vi "SourceMeterF.vi"() -> ()   [LabVIEW 2017]
uses:
  <vilib>/express/express signal manip/GetorSetDDTAttributes/Set DDT Attributes/Set DDT Properties.xnode
  <vilib>/express/express shared/transition.llb/Dynamic To Waveform Array.vi
  <vilib>/express/express signal manip/GetorSetDDTAttributes/Set DDT Attributes/SetT0.vi
  <vilib>/express/express shared/transition.llb/Waveform Array To Dynamic.vi
  <vilib>/express/express signal manip/GetorSetDDTAttributes/Set DDT Attributes/sub Set StartTimeStamp.vi
  <vilib>/express/express signal manip/GetorSetDDTAttributes/Set DDT Attributes/Set DDT Attributes.lvlib
panel:
  in  "?":bool
  in  "Registerkarte":T1(tab)
  in  "VISA resource name":refnum<visa-resource-name>
  in  "Script Name":string="myscript"
  in  "Save script (No)":bool
  in  "Load Options (Load)":enum16{"Load", "Load & Run"}(ring)
  in  "Filename":path caption="File name"
  in  "Save Data":bool
  in  "U / V":dbl=10.0
  in  "I /A":dbl=0.5
  in  "Q /C":dbl=1.0
  in  "Script":string
  out "Nr. of Measurments":i32
  out "Saving Data":bool
  out "C":dbl
  out "A":dbl
  out "V":dbl
  out "thresholdC":bool
  out "thresholdI":bool
  out "Graph":cluster{dbl, "Numerisch":dbl, "Numerisch 3":dbl}(graph)
  out "current/charge":cluster{dbl[], dbl[]}[](graph) caption="XY-Graph"
  out "Voltage":cluster{dbl[], dbl[]}(graph) caption="XY-Graph"
  out "error out 2":errorcluster
  out "current":dbl
  out "charge":dbl
  out "voltage":dbl
  out "delay1":u32
  out "delay loop2":dbl
  out "Elementanzahl in Queue":i32(slide) scale=0.0..10000.0
  # "Threshold"
  # "total time (ms)"
  # "Threshold"
  # "Threshold!"
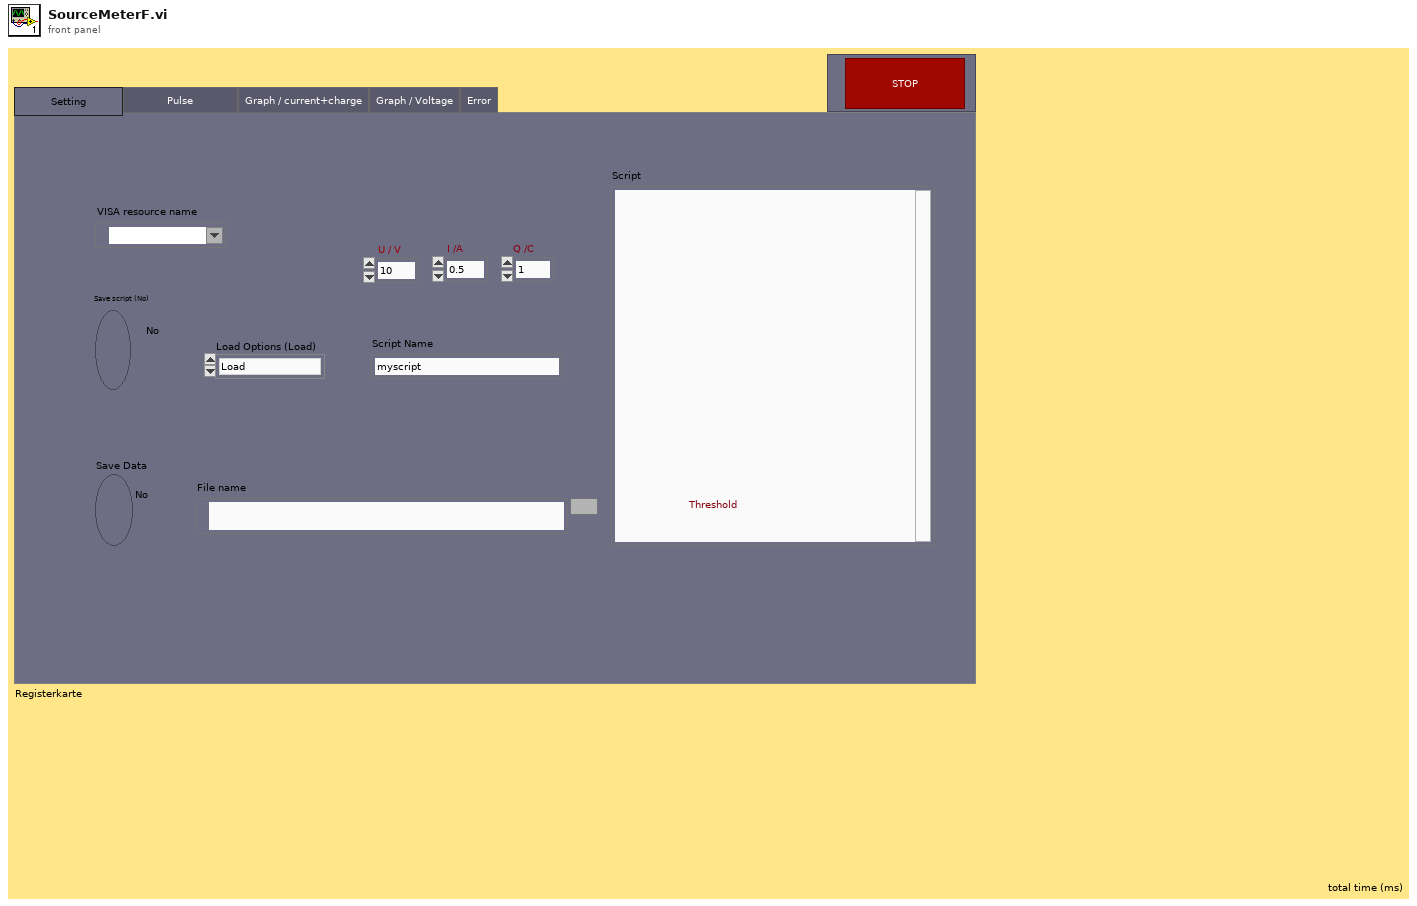
[diagram p1: front panel]
types:
  T1 = enum32{"Setting                    ", "Pulse                         ", "Graph / current+charge", "Graph / Voltage", "Error"}
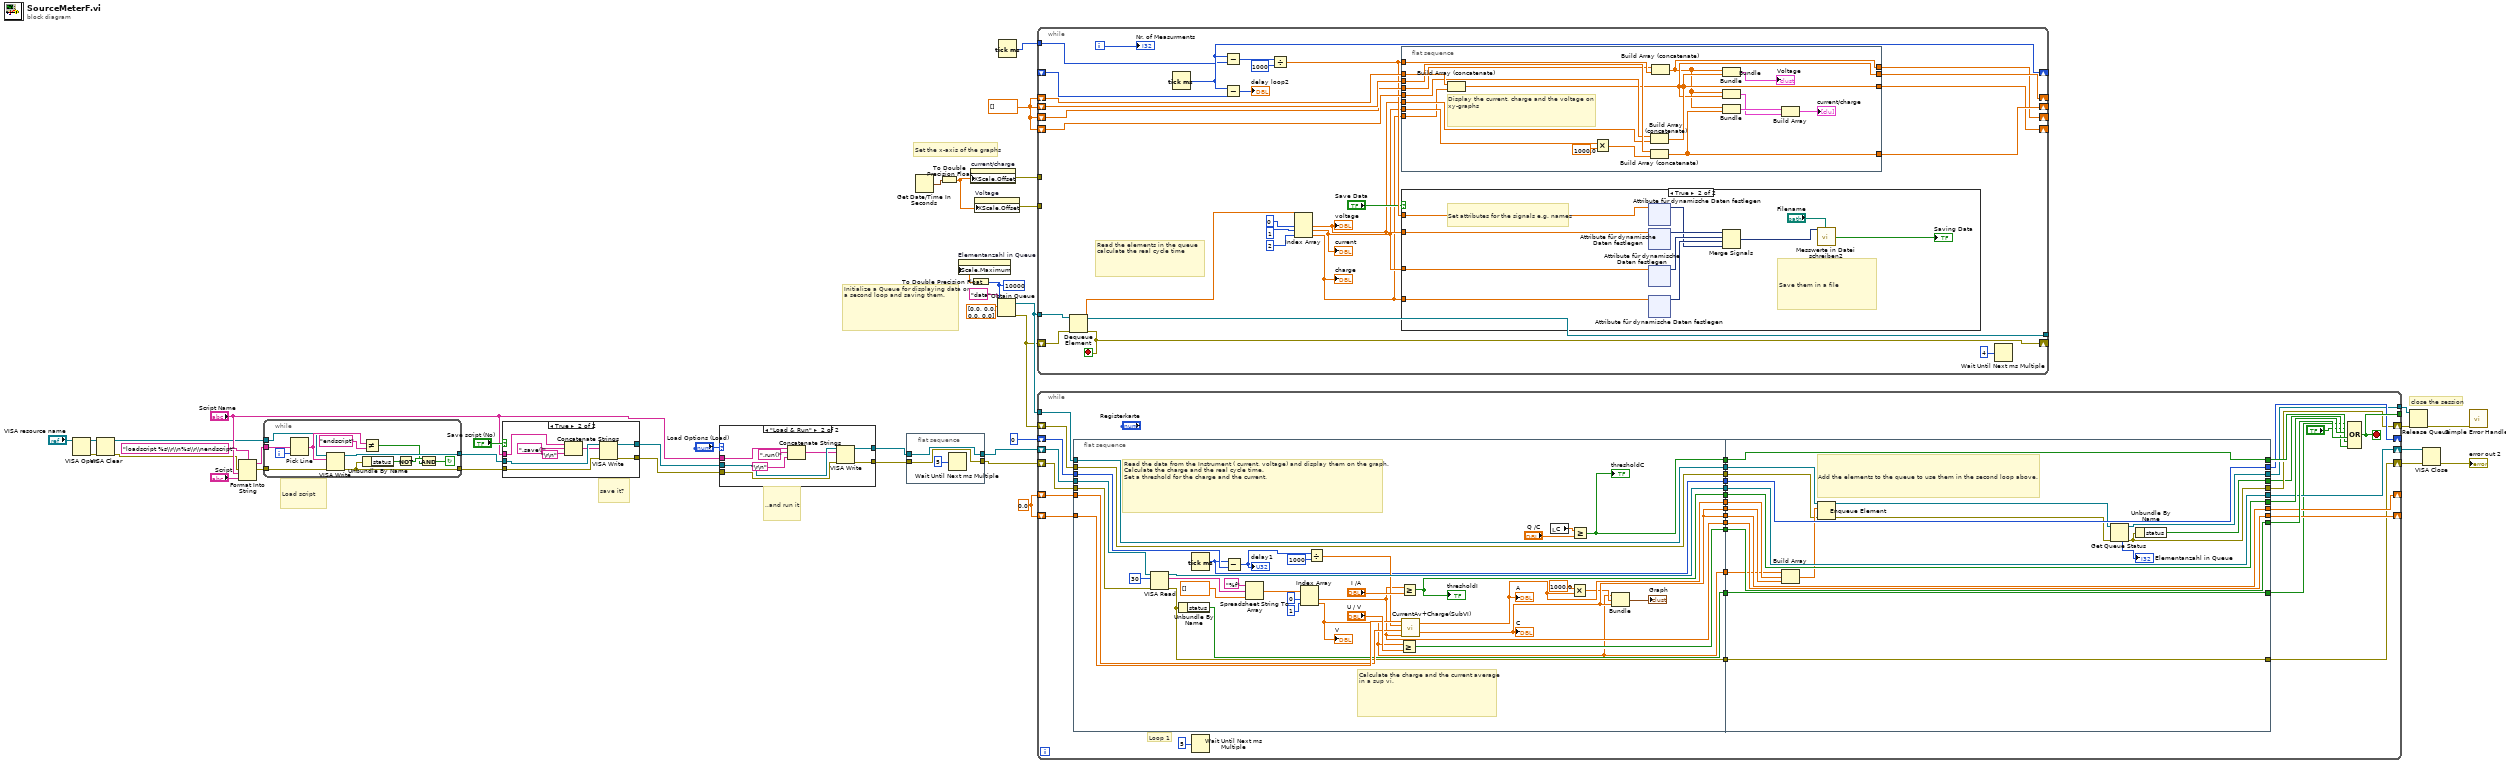
[diagram p0: block diagram]
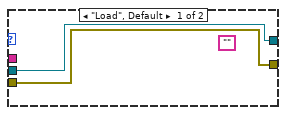
[diagram p2: hidden frame]
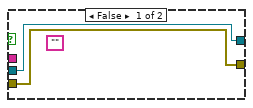
[diagram p3: hidden frame]
diagram:
  w23 = 10000 ("Maximale Queue-Größe (-1, unbegrenzt)")
  w24 = dbl[] []
  w33 = 0.0 ("Numerisch")
  # "close the session"
  # "Initialize a Queue for displaying data on a second loop and saving them."
  # "Set the x-axis of the graphs"
  # "..and run it"
  # "save it?"
  # "Load script"
  n1 = VISA Open(VISA resource name="VISA resource name") -> (VISA resource name=w20:refnum<visa-resource-name>, error out=w21:errorcluster)  [unwired: 4 in]
  n2 = VISA Clear(VISA resource name=w20, error in (no error)=w21) -> (VISA resource name out=w2:refnum<visa-resource-name>, error out=w3:errorcluster)
  n3 = Format Into String(format string="loadscript %s\\r\\n%s\\r\\nendscript", error in=w3, "Script Name", "Script") -> (resulting string=w6:string, error out=w15:errorcluster)  [unwired: 1 in]
  n4 = while {
    tunnel: w15 -> [w49]
    tunnel: [w46] -> w12
    tunnel: [w48] -> w11
    tunnel: w6 -> [w47]
    tunnel: w2 -> [w41]
    i -> [w51]
    stop <- w45 continue-if-true
    n5 = Pick Line(multi-line string=w47, line index=w51) -> (output string=w50:string)  [unwired: 1 in]
    n6 = VISA Write(VISA resource name=w41, write buffer=w50, error in (no error)=w49) -> (VISA resource name out=w48:refnum<visa-resource-name>, error out=w46:errorcluster)  [unwired: 1 out]
    n7 = Unbundle By Name(w46) -> ("status"=w44:bool)
    n8 = Not Equal?(x=w50, y="endscript") -> (x != y?=w42:bool)
    n9 = Not(x=w44) -> (.not. x?=w43:bool)
    n10 = And(x=w43, y=w42) -> (x .and. y?=w45:bool)
  }
  n11 = case shown="True" "Save script (No)" {
    tunnel: w12 -> [w53 w61]
    tunnel: w11 -> [w54 w62]
    tunnel: "Script Name" -> [_ w59]
    tunnel: [w54 w58] -> w9
    tunnel: [w53 w57] -> w8
    frame False {
      (unwired) ""
    }
    frame True {
      n12 = Concatenate Strings(w59, ".save()" ("string"), "\r\n") -> (w56:string)
      n13 = VISA Write(VISA resource name=w62, write buffer=w56, error in (no error)=w61) -> (VISA resource name out=w58:refnum<visa-resource-name>, error out=w57:errorcluster)  [unwired: 1 out]
    }
  }
  n14 = case shown="\"Load & Run\"" "Load Options (Load)" {
    tunnel: w9 -> [w64 w72]
    tunnel: w8 -> [w63 w71]
    tunnel: "Script Name" -> [_ w69]
    tunnel: [w64 w68] -> w4
    tunnel: [w63 w67] -> w5
    frame "Load", Default {
      (unwired) ""
    }
    frame "Load & Run" {
      n15 = Concatenate Strings(w69, ".run()" ("string"), "\r\n") -> (w66:string)
      n16 = VISA Write(VISA resource name=w72, write buffer=w66, error in (no error)=w71) -> (VISA resource name out=w68:refnum<visa-resource-name>, error out=w67:errorcluster)  [unwired: 1 out]
    }
  }
  n17 = flat-sequence {
    tunnel: [w74] -> w31
    tunnel: [w73] -> w32
    tunnel: w5 -> [w74]
    tunnel: w4 -> [w73]
    frame #0 {
      n18 = Wait Until Next ms Multiple(millisecond multiple=u32 5 ("Vielfache von ms")) -> ()  [unwired: 1 out]
    }
  }
  n19 = Get Date/Time In Seconds() -> (seconds since 1Jan1904=w27:timestamp)
  n20 = To Double Precision Float(number=w27) -> (double precision float=w25:dbl)
  n21 = property on="current/charge" class="XYGraph (strict)"("XScale.Offset"=w25) -> (error out=w28:errorcluster)  [unwired: 2 in, 1 out]
  n22 = To Double Precision Float(number=w23) -> (double precision float=w36:dbl)
  n23 = property on="Elementanzahl in Queue" class="Slide (strict)"("Scale.Maximum"=w36) -> ()  [unwired: 2 in, 2 out]
  n24 = property on="Voltage" class="XYGraph (strict)"("XScale.Offset"=w25) -> (error out=w26:errorcluster)  [unwired: 2 in, 1 out]
  n25 = Obtain Queue(max queue size (-1, unlimited)=w23, name (unnamed)="data" ("Name (unbenannt)"), element data type=dbl[] [0.0, 0.0, 0.0, 0.0] ("Array-Typ (2D Dbl)")) -> (queue out=w38:refnum<queue>, error out=w34:errorcluster)  [unwired: 2 in, 1 out]
  n26 = Tick Count (ms)() -> (millisecond timer value=w22:u32)
  n27 = while {
    tunnel: w38 -> [w104]
    tunnel: [w103] -> _
    shift-right: [w97] -> _
    shift-left: _ -> [w101]
    shift-right: [w100] -> _
    shift-left: w34 -> [w99]
    tunnel: w22 -> [w96]
    tunnel: w28 -> [_]
    tunnel: w26 -> [_]
    shift-right: [w88] -> _
    shift-left: w24 -> [w87]
    shift-right: [w90] -> _
    shift-left: w24 -> [w89]
    shift-right: [w92] -> _
    shift-left: w24 -> [w91]
    shift-right: [w86] -> _
    shift-left: w24 -> [w85]
    i -> [w98]
    stop <- w100 stop-if-true
    # "Read the elements in the queue\ncalculate the real cycle time"
    n28 = Dequeue Element(queue=w104, error in (no error)=w99) -> (queue out=w103:refnum<queue>, element=w102:dbl[], error out=w100:errorcluster)  [unwired: 2 out]
    n29 = Tick Count (ms)() -> (millisecond timer value=w97:u32)
    n30 = Subtract(x=w97, y=w96) -> (x-y=w94:u32)
    n31 = Subtract(x=w97, y=w101) -> (x-y=→"delay loop2":u32)
    n32 = Divide(x=w94, y=u32 1000) -> (x/y=w84:dbl)
    n33 = Index Array(array=w102, index #1=0 ("Index"), index #2=1 ("Index"), index #3=2 ("Index")) -> (element #1=w78:dbl, element #2=w77:dbl, element #3=w76:dbl)
    "voltage" <- w78
    "charge" <- w76
    "current" <- w77
    n34 = flat-sequence {
      tunnel: w78 -> [w106]
      tunnel: w77 -> [w107]
      tunnel: w76 -> [w105]
      tunnel: w84 -> [w116]
      tunnel: w91 -> [w115]
      tunnel: w89 -> [w114]
      tunnel: w87 -> [w113]
      tunnel: w85 -> [w112]
      tunnel: [w110] -> w92
      tunnel: [w109] -> w90
      tunnel: [w108] -> w88
      tunnel: [w111] -> w86
      frame #0 {
        # "Display the current, charge and the voltage on xy-graphs"
        n35 = Build Array (concatenate)(w115, w105) -> (w110:dbl[])
        n36 = Multiply(x=w107, y=1000.0 ("x")) -> (x*y=w117:dbl)
        n37 = Build Array (concatenate)(w112, w106) -> (w111:dbl[])
        n38 = Build Array (concatenate)(w114, w117) -> (w109:dbl[])
        n39 = Build Array (concatenate)(w113, w116) -> (w108:dbl[])
        n40 = Bundle(w108, w111) -> (→"Voltage":cluster{dbl[], dbl[]})  [unwired: 1 in]
        n41 = Bundle(w108, w110) -> (w120:cluster{dbl[], dbl[]})  [unwired: 1 in]
        n42 = Bundle(w108, w109) -> (w121:cluster{dbl[], dbl[]})  [unwired: 1 in]
        n43 = Build Array(w121, w120) -> (→"current/charge":cluster{dbl[], dbl[]}[])
      }
    }
    n44 = case shown="True" "Save Data" {
      tunnel: w78 -> [_ w133]
      tunnel: w76 -> [_ w132]
      tunnel: w77 -> [_ w131]
      tunnel: w84 -> [_ w130]
      frame False {
      }
      frame True {
        # "Set attributes for the signals e.g. names"
        # "Save them in a file"
        n45 = xnode ("Attribute für dynamische Daten festlegen")("Signals In"=w130) -> ("Signals Out"=w125:dynamicdata)  [unwired: 3 in, 1 out]
        n46 = xnode ("Attribute für dynamische Daten festlegen")("Signals In"=w133) -> ("Signals Out"=w128:dynamicdata)  [unwired: 3 in, 1 out]
        n47 = xnode ("Attribute für dynamische Daten festlegen")("Signals In"=w131) -> ("Signals Out"=w127:dynamicdata)  [unwired: 3 in, 1 out]
        n48 = xnode ("Attribute für dynamische Daten festlegen")("Signals In"=w132) -> ("Signals Out"=w126:dynamicdata)  [unwired: 4 in, 1 out]
        n49 = Merge Signals(w128, w127, w126, w125) -> (w129:dynamicdata)
        n50 = call "Messwerte in Datei schreiben2"("Signals"=w129, "Filename"="Filename") -> ("Saving Data"=→"Saving Data":bool)  [unwired: 15 in, 2 out]
      }
    }
    n51 = Wait Until Next ms Multiple(millisecond multiple=u32 4) -> ()  [unwired: 1 out]
    "Nr. of Measurments" <- w98
  }
  n52 = while {
    shift-right: [w224] -> _
    shift-left: w33 -> [w227]
    shift-right: [w225] -> _
    shift-left: w33 -> [w226]
    tunnel: w38 -> [w205]
    tunnel: [w223] -> _
    shift-right: [w201] -> w35
    shift-left: w34 -> [w203]
    shift-right: [w220] -> w18
    shift-left: w32 -> [w218]
    shift-right: [w219] -> w19
    shift-left: w31 -> [w217]
    shift-right: [w215] -> _
    shift-left: u32 0 ("millisecond timer value") -> [w216]
    tunnel: [w199] -> w29
    stop <- w223 stop-if-true
    # "Loop 1"
    n53 = flat-sequence {
      tunnel: w227 -> [w259]
      tunnel: w226 -> [w258]
      tunnel: w218 -> [w231]
      tunnel: w217 -> [w232]
      tunnel: w216 -> [w250]
      tunnel: [w260] -> w214
      tunnel: [w244] -> w213
      tunnel: [w234] -> w212
      tunnel: [w255] -> w211
      tunnel: [w254] -> w210
      tunnel: [w253] -> w209
      tunnel: [w252] -> w208
      tunnel: [w251] -> w207
      tunnel: [w229] -> w206
      tunnel: w205 -> [w246]
      tunnel: [w246] -> w204
      tunnel: w203 -> [w245]
      tunnel: [w245] -> w202
      tunnel: [w244] -> w198
      tunnel: [w243] -> w197
      tunnel: [w233] -> w196
      tunnel: [w276] -> w215
      tunnel: [w277] -> w219
      tunnel: [w278] -> w220
      tunnel: [w279] -> w221
      tunnel: [w280] -> w222
      tunnel: [w281] -> w193
      tunnel: [w282] -> w224
      tunnel: [w283] -> w225
      tunnel: [w284] -> w228
      tunnel: w214 -> [w284]
      tunnel: w213 -> [w283]
      tunnel: w212 -> [w282]
      tunnel: w211 -> [w281]
      tunnel: w210 -> [w280]
      tunnel: w209 -> [w279]
      tunnel: w208 -> [w278]
      tunnel: w207 -> [w277]
      tunnel: w206 -> [w276]
      tunnel: w204 -> [w271]
      tunnel: w202 -> [w270]
      tunnel: [w269] -> w200
      tunnel: [w268] -> w201
      tunnel: [w267] -> w199
      tunnel: w198 -> [w266]
      tunnel: w197 -> [w265]
      tunnel: w196 -> [w264]
      frame #0 {
        # "Calculate the charge and the current average\nin a sup vi."
        # "Read the data from the Instrument ( current, voltage) and display them on the graph.\nCalculate the charge and the real cycle time.\nSet a threshold for the charge and the current."
        n54 = VISA Read(VISA resource name=w231, byte count=u32 30 ("Byte-Anzahl"), error in (no error)=w232) -> (VISA resource name out=w252:refnum<visa-resource-name>, read buffer=w240:string, error out=w251:errorcluster)  [unwired: 1 out]
        n55 = Unbundle By Name(w251) -> ("status"=w255:bool)
        n56 = Tick Count (ms)() -> (millisecond timer value=w229:u32)
        n57 = Subtract(x=w229, y=w250) -> (x-y=w249:u32)
        "delay1" <- w249
        n58 = Spreadsheet String To Array(format string="%f" ("Format-String"), spreadsheet string=w240, array type (2D Dbl)=dbl[] [] ("Array-Typ (2D Dbl)")) -> (array=w237:dbl[])  [unwired: 1 in]
        n59 = Index Array(array=w237, index #1=0 ("Index"), index #2=1 ("Index")) -> (element #1=w234:dbl, element #2=w233:dbl)
        "V" <- w233
        n60 = Divide(x=w249, y=u32 1000) -> (x/y=w247:dbl)
        n61 = Greater Or Equal?(x=w233, y="U / V") -> (x >= y?=w260:bool)
        n62 = Greater Or Equal?(x=w234, y="I /A") -> (x >= y?=w253:bool)
        "thresholdI" <- w253
        n63 = call "CurrentAv+Charge(SubVI).vi"("current 0"=w234, "charge 0"=w258, "measureRate"=w247, "current"=w259) -> ("charge"=w244:dbl, "current Av."=w243:dbl)
        "C" <- w244
        "A" <- w243
        n64 = local read "C"() -> (w256:dbl)
        n65 = Multiply(x=1000.0, y=w243) -> (x*y=w242:dbl)
        n66 = Greater Or Equal?(x=w256, y="Q /C") -> (x >= y?=w254:bool)
        "thresholdC" <- w254
        n67 = Bundle(w233, w242, "charge"=w244) -> (→"Graph":cluster{dbl, dbl, "charge":dbl})  [unwired: 1 in]
      }
      frame #1 {
        # "Add the elements to the queue to use them in the second loop above."
        n68 = Build Array(w264, w265, w266) -> (w272:dbl[])
        n69 = Enqueue Element(queue=w271, element=w272, error in (no error)=w270) -> (queue out=w274:refnum<queue>, error out=w273:errorcluster)  [unwired: 2 out]
        n70 = Get Queue Status(queue=w274, error in (no error)=w273) -> (queue out=w267:refnum<queue>, error out=w268:errorcluster, # elements in queue=→"Elementanzahl in Queue":i32)  [unwired: 6 out]
        n71 = Unbundle By Name(w268) -> ("status"=w269:bool)
      }
    }
    n72 = Wait Until Next ms Multiple(millisecond multiple=u32 5) -> ()  [unwired: 1 out]
    n73 = Compound Arithmetic op=OR(w193, "?", w221, w228, w222, w200) -> (w223:bool)
  }
  n74 = Release Queue(queue=w29, error in (no error)=w35) -> (error out=w37:errorcluster)  [unwired: 3 out]
  n75 = VISA Close(VISA resource name=w18, error in (no error)=w19) -> (error out=→"error out 2":errorcluster)
  n76 = call <vilib>:"Simple Error Handler.vi"("error in (no error)"=w37) -> ()  [unwired: 1 in, 8 out]
